vi "Get lvclass files in subfolder.vi"(8 "Error In":errorcluster, 11 "Sub Folder":string) -> (0 "Error Out":errorcluster, 3 "Found lvclass files":path[](array[path]))   [LabVIEW 2020]
doc: "Finds all LVCLASS files in subfolder of the application"
panel:
  out "size(s)":i32
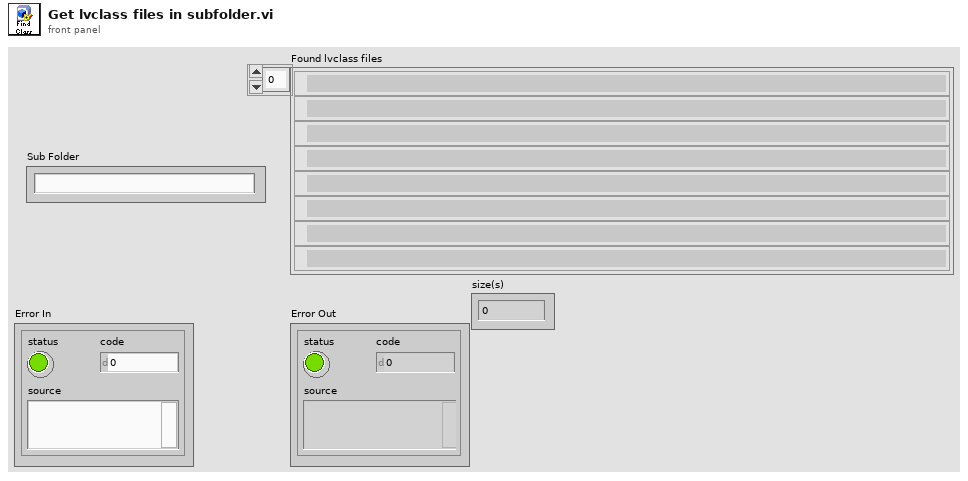
[diagram p1: front panel]
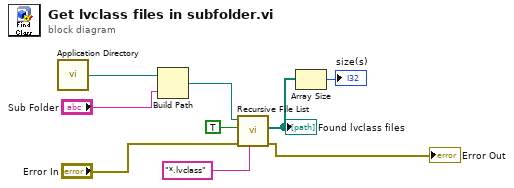
[diagram p0: block diagram]
diagram:
  n1 = call <vilib>:"Application Directory.vi"() -> ("Application Directory"=w9:path)
  n2 = Build Path(base path=w9, name or relative path="Sub Folder") -> (appended path=w7:path)
  n3 = call <vilib>:"Recursive File List.vi"("pattern"="*.lvclass", "error in (no error)"="Error In", "Treat LLBs as Folders?"=TRUE, "Folder Path"=w7) -> ("error out"=→"Error Out":errorcluster, "All Files in Dir"=w2:path[])  [unwired: 3 in, 3 out]
  "Found lvclass files" <- w2
  n4 = Array Size(array=w2) -> (size(s)=→"size(s)":i32)
